vi "BotSpeak_RIO_TextDisplay.vi"(2 "Position":cluster{"Row":u8, "Col":u8}, 3 "Text":string="Test", 4 "Bot Settings":T1) -> (1 "Bot Settings 2":T1)   [LabVIEW 2012]
doc: "Displays text to the RIO's Screen. Takes in the desired \"Text\" as a string, and places it according to the cluster of two values indicating \"Position\"."
uses:
  <userlib>/BotSpeak/VIs/Direct/BotSpeak_Control.ctl
panel:
  out "response":string="169.254.32.85"
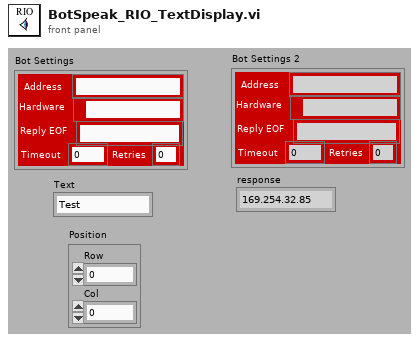
[diagram p1: front panel]
types:
  T1 = typedef "BotSpeak_Control.ctl" = cluster{"Address":string, "Reply EOF":string, "Hardware":path, "Retries":i8, "Timeout":i32}
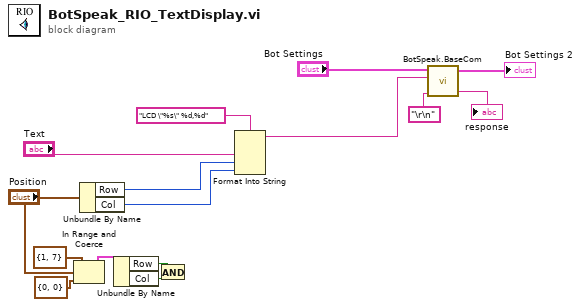
[diagram p0: block diagram]
diagram:
  n1 = In Range and Coerce(upper limit=cluster{"Row":u8, "Col":u8} {"Row"=1, "Col"=7}, x="Position", lower limit=cluster{"Row":u8, "Col":u8} {"Row"=0, "Col"=0} ("upper limit")) -> (In Range?=w8:cluster{"Row":bool, "Col":bool})  [unwired: 1 out]
  n2 = Unbundle By Name("Position") -> ("Row"=w13:u8, "Col"=w12:u8)
  n3 = Unbundle By Name(w8) -> ("Row"=w6:bool, "Col"=w7:bool)
  n4 = And(x=w6, y=w7) -> ()  [unwired: 1 out]
  n5 = Format Into String(format string="LCD \"%s\" %d,%d" ("command"), "Text", w13, w12) -> (resulting string=w1:string)  [unwired: 2 in, 1 out]
  n6 = call <userlib>:"BotSpeak.BaseCom.vi"("Termination"="\r\n", "command"=w1, "Bot Settings in"="Bot Settings") -> ("response"=→"response":string, "Bot Settings out"=→"Bot Settings 2":T1)  [unwired: 2 in]
